vi "Main.vi"(11 "Module Admin":refnum<class "Delacor_lib_QMH_Module Admin.lvclass">) -> ()   [LabVIEW 2024, in "IOLink.lvlib"]
doc: "This template is based off of the Queued Message Handler design pattern and the Queued Message Handler project template that ships with LabVIEW.\n\nThe main difference is that the queue is private to this module and communication between modules is performed via Broadcast and Request events.\n\nRequest events are wrapped in public API methods and are handled in the Event Handling Loop (EHL) of this VI. Any module can register for Broadcast events sent by this module. The EHL generates messages based on user interface actions.\n\nThe Message Handling Loop (MHL) processes messages generated by the EHL, or by other messages. The messages are string values, so new messages can be added easily to the Message Cases case structure in the MHL. Each message cluster can also provide an optional value for Message Data, which is a variant that can be converted to whatever message-specific data is required.\n_____\nBased on DQMH Project Template 7.0.0.1280."
uses:
  IOLink.lvlib
  <vilib>/Delacor/Delacor QMH/Libraries/Module Admin_class/Delacor_lib_QMH_Module Admin.lvclass
  Module Data--cluster.ctl
  <vilib>/NI/Modbus Library/API/Master/Modbus Master.lvclass
  Start IOL Data Acquisition (Reply Payload)--cluster.ctl
  <vilib>/Delacor/Delacor QMH/Libraries/Message Queue_class/Delacor_lib_QMH_Message Queue.lvclass/Delacor_lib_QMH_Message Queue.ctl
  Stop Argument--cluster.ctl
  <vilib>/Delacor/Delacor QMH/Libraries/Module Admin_class/Delacor_lib_QMH_Module Admin.lvclass/Delacor_lib_QMH_Module Admin.ctl
  <vilib>/Utility/miscctls.llb/LVPointTypeDef.ctl
  <vilib>/Delacor/Delacor QMH/Libraries/Message Queue_class/Delacor_lib_QMH_Enqueue Message (Single).vi
  <vilib>/Delacor/Delacor QMH/Libraries/Module Admin_class/Delacor_lib_QMH_Get External Launch.vi
  <vilib>/NI/Modbus Library/API/Wrapper/Create TCP Master.vi
  <vilib>/Delacor/Delacor QMH/Libraries/Message Queue_class/Delacor_lib_QMH_Message Queue.lvclass
  <vilib>/NI/Modbus Library/API/Wrapper/API Main.lvlib
panel:
  out "map out":map{string, dbl}(c390)
  out "X5-8 Invalid Data":bool[](array[boolean])
  out "X5-8 Not Connected":bool[](array[boolean])
  out "X1-4 Invalid Data":bool[](array[boolean])
  out "X1-4 Not Connected":bool[](array[boolean])
  out "error out":errorcluster
  out "Status":string
  in  "Simulate MHL Error":bool
  in  "Simulate EHL Error":bool
  # "This template is for the DQMH framework. See the block diagram for more information on how to use this template."
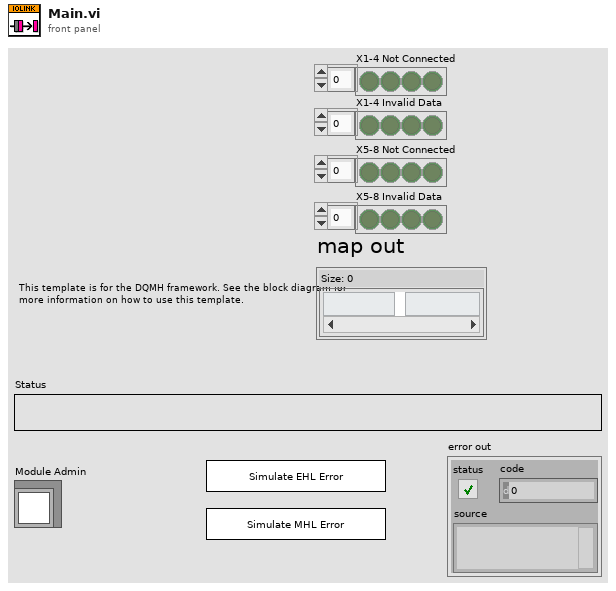
[diagram p1: front panel]
types:
  T1 = typedef "IOLink.lvlib/Request Events--cluster.ctl" = cluster{"Stop Module":refnum<user-event>, "Show Panel":refnum<user-event>, "Hide Panel":refnum<user-event>, "Get Module Execution Status":refnum<user-event>, "Show Diagram":refnum<user-event>, "Start IOL Data Acquisition":refnum<user-event>}
  T2 = typedef "IOLink.lvlib/Module Data--cluster.ctl" = cluster{"Status":string, "TCP master instance":refnum<class "Modbus Master.lvclass">}
  T3 = typedef "IOLink.lvlib/Start IOL Data Acquisition (Reply Payload)--cluster.ctl" = cluster{"error":errorcluster}
  T4 = enum32{"invalid lock state", "Not Locked", "Locked (No Password)", "Password-protected"}
  T5 = typedef "IOLink.lvlib/Stop Argument--cluster.ctl" = cluster{"Origin":string, "Exit via Stop Module Req?":bool, "Wait for Module to stop?":bool}
  T6 = typedef "LVPointTypeDef.ctl" = cluster{"Horizontal":i16, "Vertical":i16}
  T7 = enum32{"Invalid", "Standard", "Closed", "Hidden", "Minimized", "Maximized"}
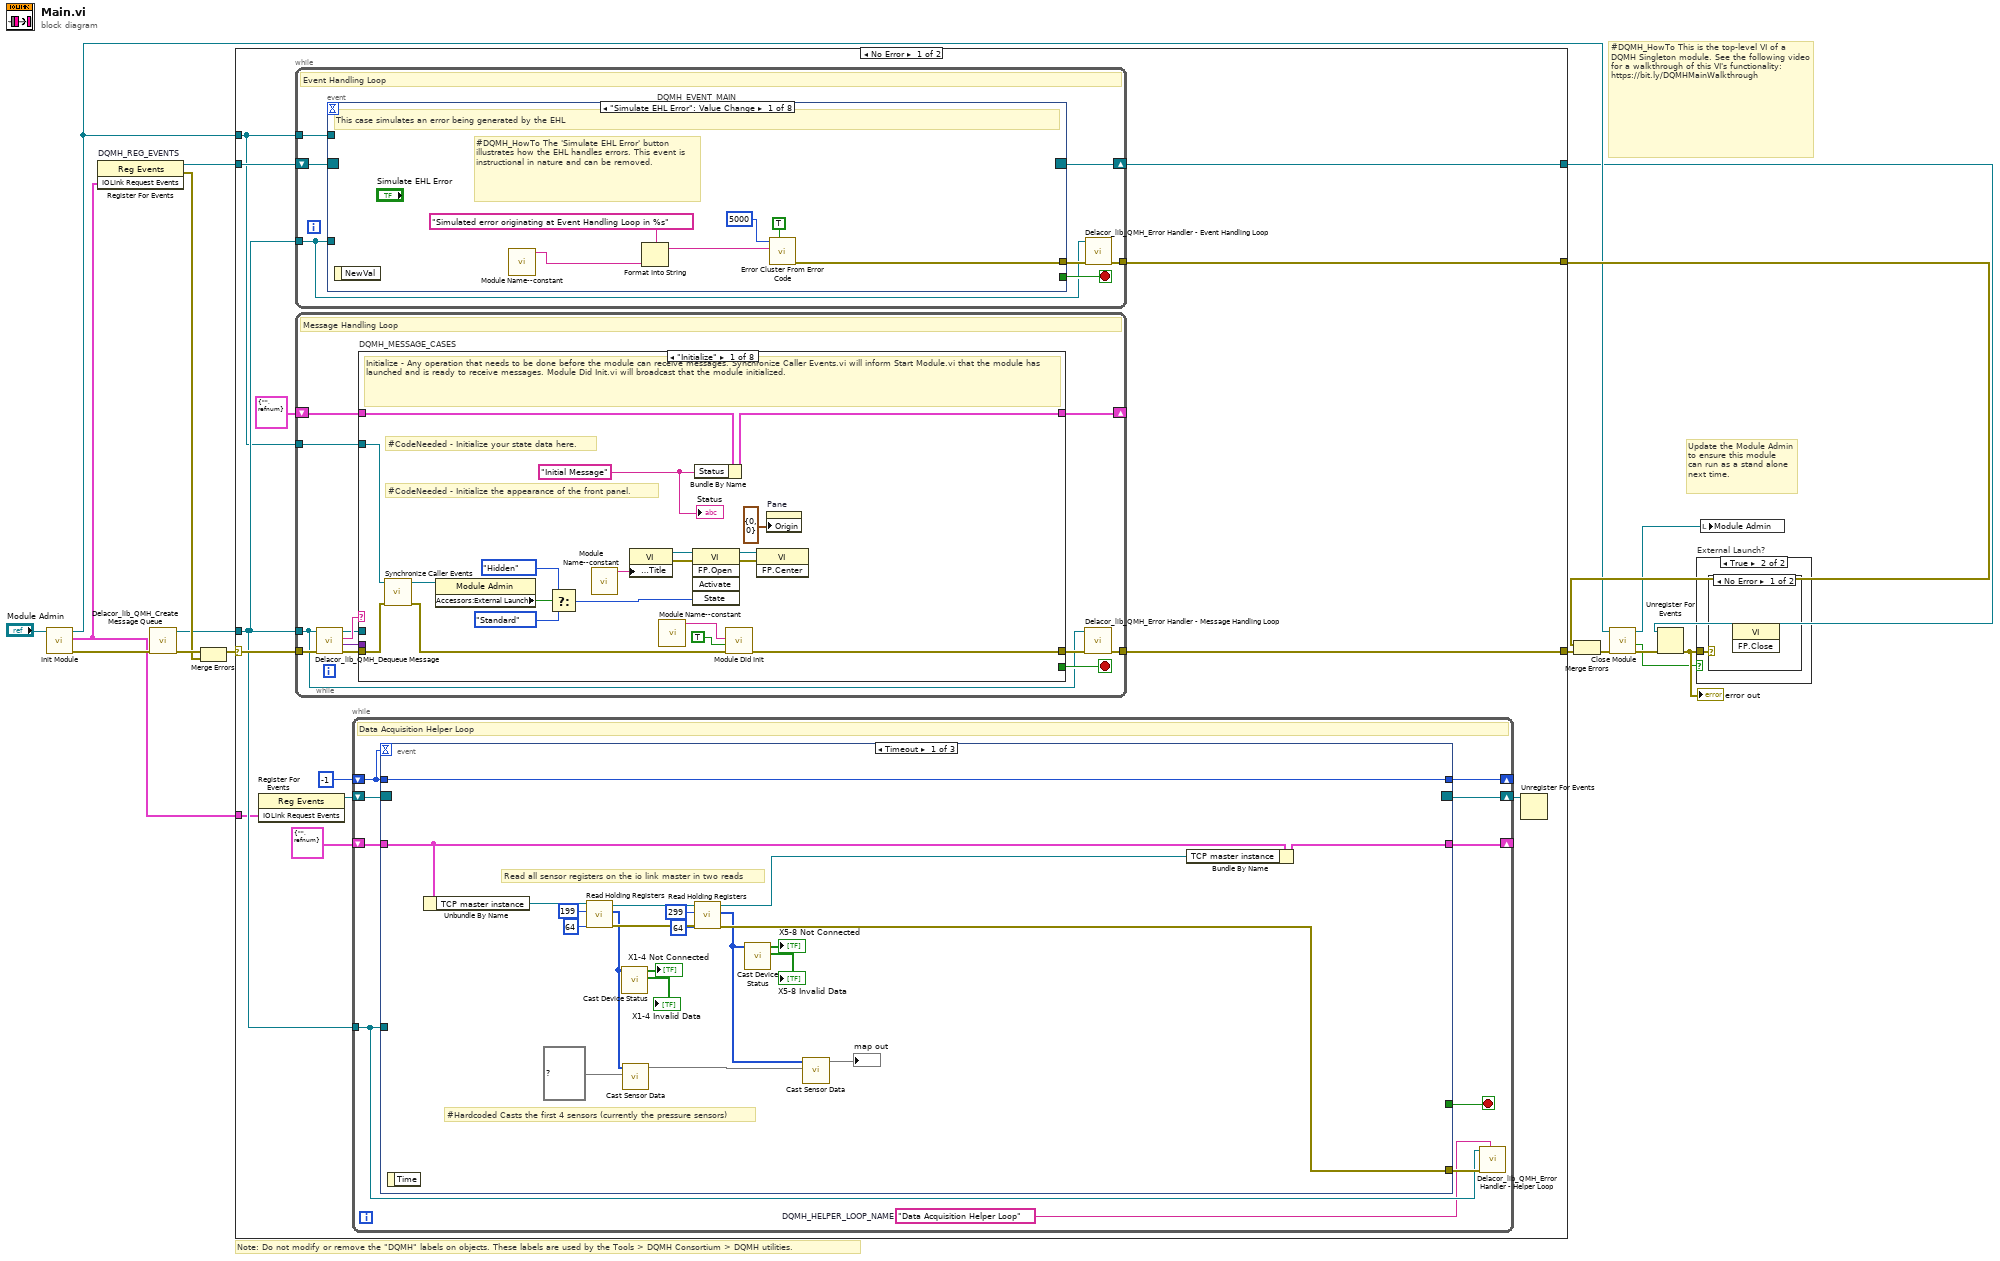
[diagram p0: block diagram]
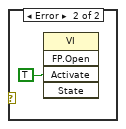
[diagram p3: hidden frame]
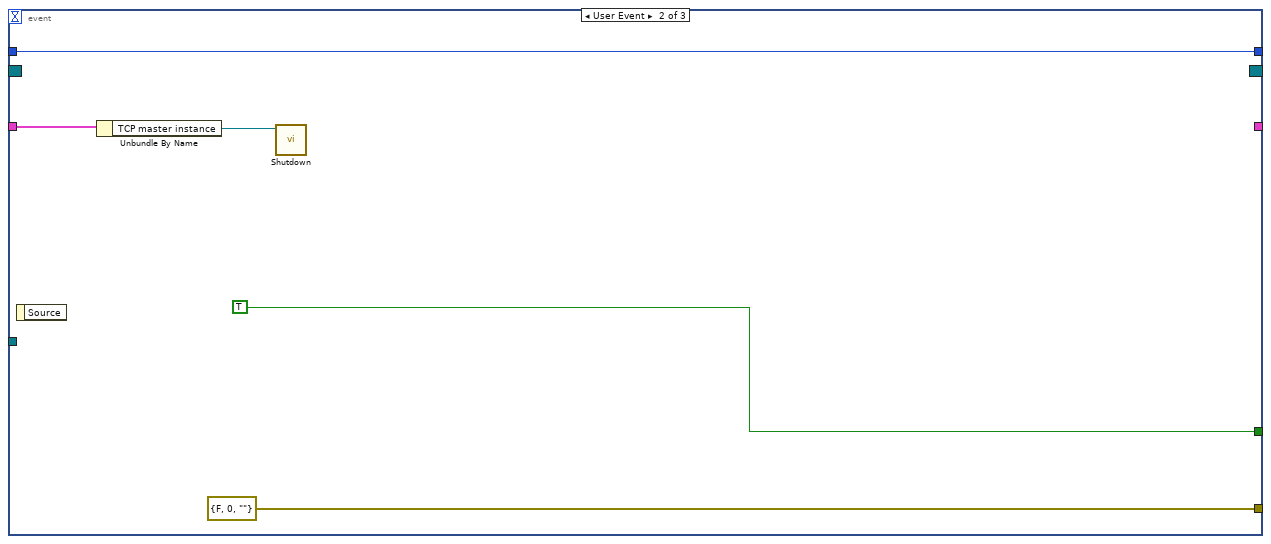
[diagram p4: hidden frame]
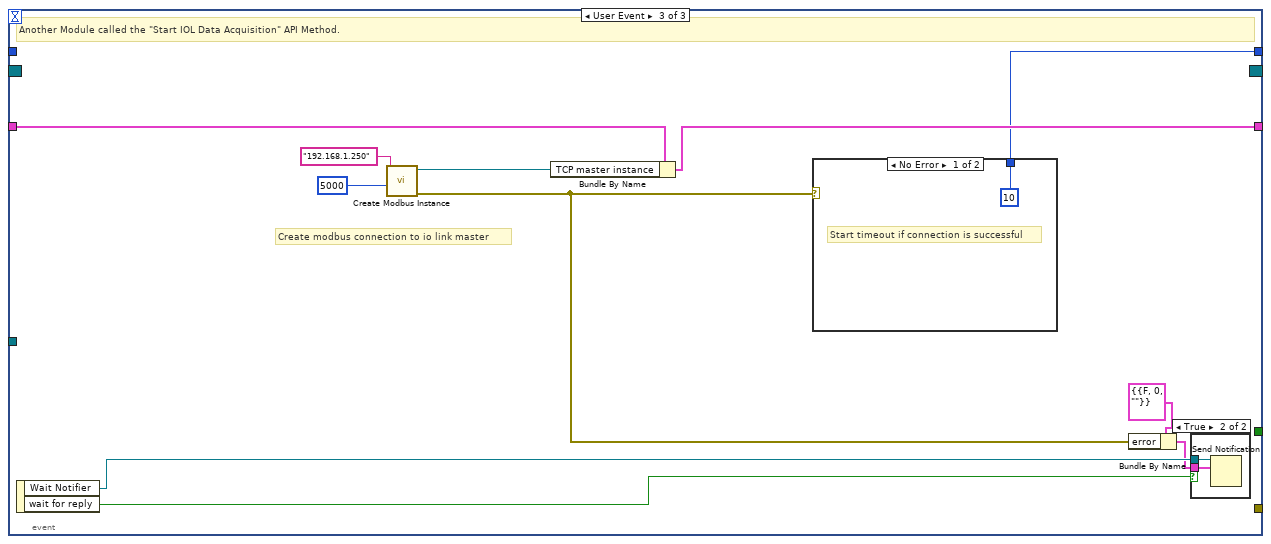
[diagram p5: hidden frame]
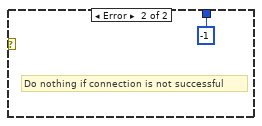
[diagram p6: hidden frame]
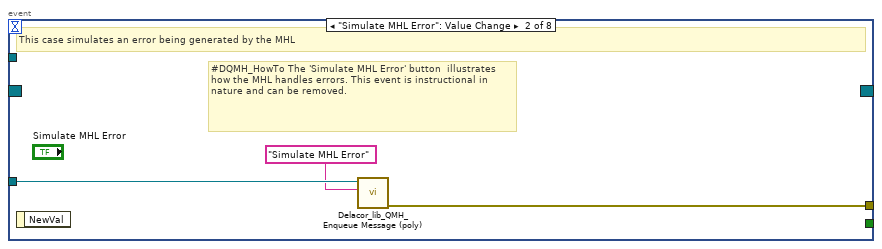
[diagram p8: hidden frame]
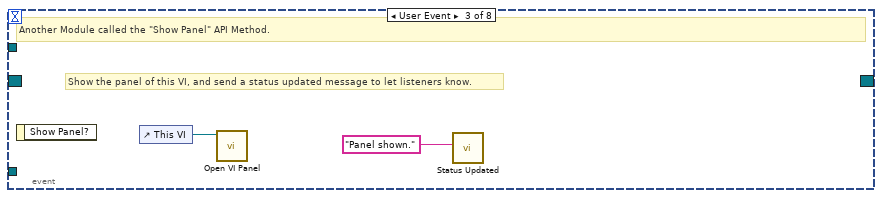
[diagram p9: hidden frame]
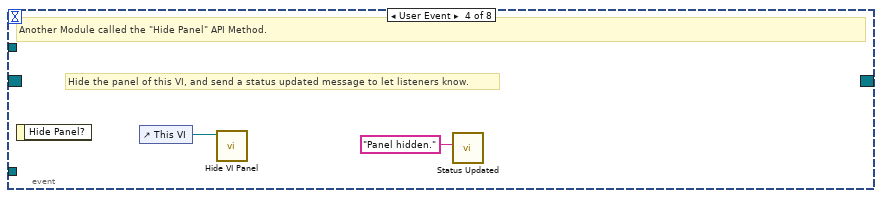
[diagram p10: hidden frame]
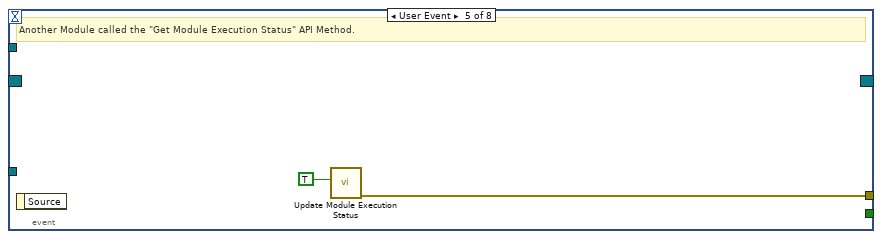
[diagram p11: hidden frame]
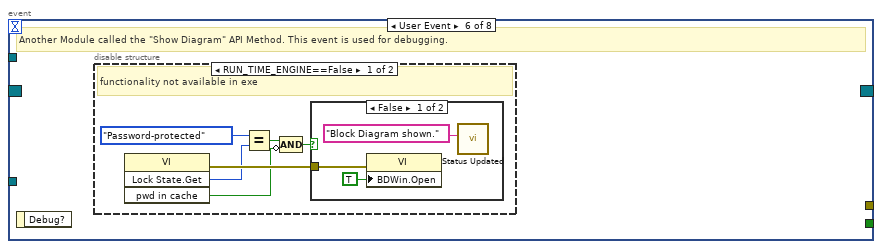
[diagram p12: hidden frame]
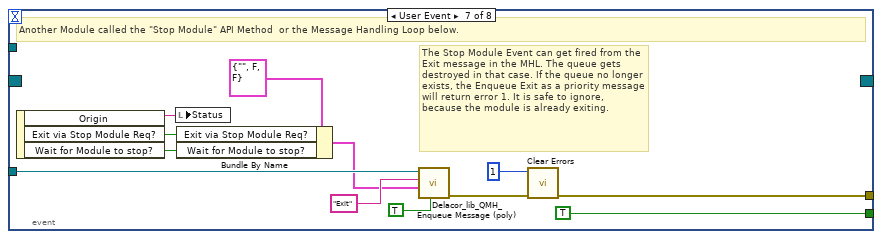
[diagram p15: hidden frame]
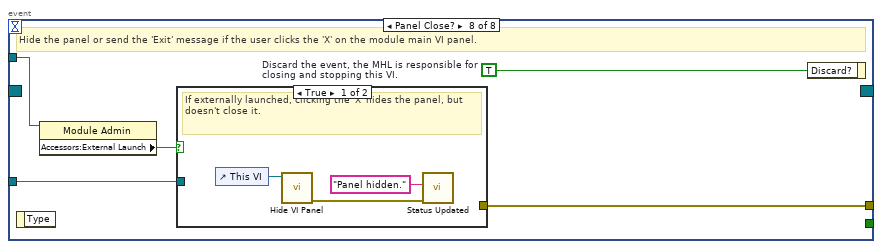
[diagram p16: hidden frame]
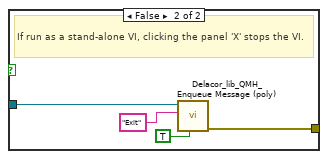
[diagram p17: hidden frame]
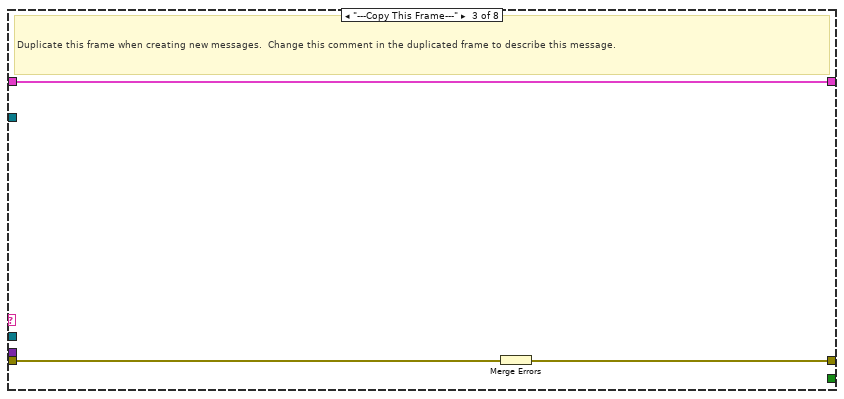
[diagram p19: hidden frame]
diagram:
  # "#DQMH_HowTo This is the top-level VI of a DQMH Singleton module. See the following video for a walkthrough of this VI's functionality: https://bit.ly/DQMHMainWalkthrough"
  # "Note: Do not modify or remove the \"DQMH\" labels on objects. These labels are used by the Tools > DQMH Consortium > DQMH utilities."
  # "Update the Module Admin to ensure this module can run as a stand alone next time."
  n1 = call "Init Module.vi"("Singleton Module Admin in"="Module Admin") -> ("error out"=w16:errorcluster, "IOLink Request Events"=w1:T1, "Singleton Module Admin out"=w8:refnum<class "Delacor_lib_QMH_Module Admin.lvclass">)  [unwired: 8 in]
  n2 = register-events "DQMH_REG_EVENTS"(w1) -> (reference out=w6:refnum<event-registration>, error out=w9:errorcluster)  [unwired: 2 in]
  n3 = call <vilib>:"Delacor_lib_QMH_Create Message Queue.vi"("error in"=w16) -> ("error out"=w11:errorcluster, "Message Queue"=w5:refnum<class "Delacor_lib_QMH_Message Queue.lvclass">)  [unwired: 9 in]
  n4 = Merge Errors(w11, w9) -> (w10:errorcluster)
  n5 = case shown="No Error" w10 {
    selector: w10 -> [w28 w234]
    tunnel: [w30 w233] -> w17
    tunnel: [w27 w232] -> w7
    tunnel: w6 -> [w25 w232]
    tunnel: w5 -> [w24 w227]
    tunnel: [w29 _] -> w14
    tunnel: w8 -> [w23 w228]
    tunnel: w1 -> [w22 _]
    frame No Error {
      n6 = register-events ("DQMH_HELPER_REGFOREVENTS")(w22) -> (reference out=w20:refnum<event-registration>)  [unwired: 2 in, 1 out]
      n7 = while {
        tunnel: w24 -> [w82]
        shift-right: [w85] -> w27
        shift-left: w25 -> [w86]
        tunnel: [w87] -> w29
        tunnel: w23 -> [w83]
        stop <- w84 stop-if-true
        # "Event Handling Loop"
        n8 = event "DQMH_EVENT_MAIN" shown="[0] \"Simulate EHL Error\": Value Change" {
          selector: w86 -> [_ _ _ _ _ _ _ _]
          dyn-events: [_ _ _ _ _ _ _ _] -> w85
          timeout: _ -> [_ _ _ _ _ _ _ _]
          tunnel: [_ _ _ _ _ _ TRUE ("Discard?") _] -> w84
          tunnel: w82 -> [_ w96 _ _ _ _ w120 w127]
          tunnel: [w94 w97 _ _ w103 _ w123 w129] -> w88
          tunnel: w83 -> [_ _ _ _ _ _ _ w126]
          event "Simulate EHL Error": Value Change {
            # "#DQMH_HowTo The 'Simulate EHL Error' button  illustrates how the EHL handles errors. This event is instructional in nature and can be removed."
            # "This case simulates an error being generated by the EHL"
            n9 = event-data() -> ()  [unwired: 1 in, 1 out]
            n10 = call "Module Name--constant.vi"() -> ("Module Name"=w91:string)  [unwired: 11 in]
            n11 = Format Into String(format string="Simulated error originating at Event Handling Loop in %s", w91) -> (resulting string=w92:string)  [unwired: 2 in, 1 out]
            n12 = call <vilib>:"Error Cluster From Error Code.vi"("show call chain? (False)"=TRUE, "error message (\"\")"=w92, "error code (0)"=5000) -> ("error out"=w94:errorcluster)  [unwired: 6 in]
          }
          event "Simulate MHL Error": Value Change {
            # "#DQMH_HowTo The 'Simulate MHL Error' button  illustrates how the MHL handles errors. This event is instructional in nature and can be removed."
            # "This case simulates an error being generated by the MHL"
            n13 = event-data() -> ()  [unwired: 1 in, 1 out]
            n14 = call-poly <vilib>:"Delacor_lib_QMH_Enqueue Message (poly).vi"("Message"="Simulate MHL Error", "Message Queue in"=w96) -> ("error out"=w97:errorcluster)  [unwired: 8 in, 1 out]
          }
          event User Event {
            # "Show the panel of this VI, and send a status updated message to let listeners know."
            # "Another Module called the \"Show Panel\" API Method."
            n15 = event-data() -> ()  [unwired: 1 in, 1 out]
            n16 = control-ref of="This VI"() -> (w99:refnum<vi>)
            n17 = call "Open VI Panel.vi"("VI"=w99) -> ()  [unwired: 10 in, 1 out]
            n18 = call "Status Updated.vi"("Status"="Panel shown." ("format string")) -> ()  [unwired: 10 in, 1 out]
          }
          event User Event {
            # "Hide the panel of this VI, and send a status updated message to let listeners know."
            # "Another Module called the \"Hide Panel\" API Method."
            n19 = event-data() -> ()  [unwired: 1 in, 1 out]
            n20 = control-ref of="This VI"() -> (w101:refnum<vi>)
            n21 = call "Hide VI Panel.vi"("VI"=w101) -> ()  [unwired: 10 in, 1 out]
            n22 = call "Status Updated.vi"("Status"="Panel hidden." ("format string")) -> ()  [unwired: 10 in, 1 out]
          }
          event User Event {
            # "Another Module called the \"Get Module Execution Status\" API Method."
            n23 = event-data() -> ()  [unwired: 1 in, 1 out]
            n24 = call "Update Module Execution Status.vi"("Running?"=TRUE) -> ("error out"=w103:errorcluster)  [unwired: 10 in]
          }
          event User Event {
            # "Another Module called the \"Show Diagram\" API Method. This event is used for debugging."
            n25 = event-data() -> ()  [unwired: 1 in, 1 out]
            n26 = disable-structure shown="RUN_TIME_ENGINE==False" {
              frame condition #0 (active) {
                # "functionality not available in exe"
                n27 = invoke class="VI" method="Lock State.Get"() -> (error out=w109:errorcluster, "Get Lock State"=w108:T4, "pwd in cache"=w105:bool)  [unwired: 4 in, 1 out]
                n28 = Equal?(x=T4."Password-protected", y=w108) -> (x = y?=w106:bool)
                n29 = Compound Arithmetic op=AND(w106, invert w105) -> (w104:bool)
                n30 = case shown="False" w104 {
                  tunnel: w109 -> [w112 _]
                  frame False {
                    n31 = property class="VI"(error in=w112, "BDWin.Open"=TRUE ("Block Diagram Window:Open")) -> ()  [unwired: 1 in, 2 out]
                    n32 = call "Status Updated.vi"("Status"="Block Diagram shown." ("format string")) -> ()  [unwired: 10 in, 1 out]
                  }
                  frame True {
                    # "Password-protected VI, and the password is not in the cache. Do not show the diagram."
                  }
                }
              }
              frame condition #1 {
              }
            }
          }
          event User Event {
            # "The Stop Module Event can get fired from the Exit message in the MHL. The queue gets destroyed in that case. If the queue no longer exists, the Enqueue Exit as a priority message will return error 1. It is safe to ignore, because the module is already exiting."
            # "Another Module called the \"Stop Module\" API Method  or the Message Handling Loop below."
            n33 = event-data() -> ("Origin"=w119:string, "Exit via Stop Module Req?"=w115:bool, "Wait for Module to stop?"=w114:bool)  [unwired: 1 in]
            n34 = local write "Status"(w119) -> ()
            n35 = Bundle By Name(cluster=T5 {"Origin"="", "Exit via Stop Module Req?"=FALSE, "Wait for Module to stop?"=FALSE} ("Stop Argument"), "Exit via Stop Module Req?"=w115, "Wait for Module to stop?"=w114) -> (w113:T5)
            n36 = call-poly <vilib>:"Delacor_lib_QMH_Enqueue Message (poly).vi"("Priority Message? (F)"=TRUE, "Message Data"=w113, "Message"="Exit", "Message Queue in"=w120) -> ("error out"=w124:errorcluster)  [unwired: 6 in, 1 out]
            n37 = call <vilib>:"Clear Errors.vi"("error in (no error)"=w124, "specific error code to clear (0: all)"=1) -> ("error out"=w123:errorcluster)  [unwired: 4 in, 1 out]
          }
          event Panel Close? {
            w128 = TRUE  # Discard the event, the MHL is responsible for closing and stopping this VI.
            # "Hide the panel or send the 'Exit' message if the user clicks the 'X' on the module main VI panel."
            n38 = event-data() -> ()  [unwired: 1 in, 1 out]
            n39 = property class="Module Admin"(reference=w126) -> ("Accessors:External Launch"=w125:bool)  [unwired: 1 in, 2 out]
            n40 = case shown="True" w125 {
              tunnel: w127 -> [_ w135]
              tunnel: [_ w136] -> w129
              frame True {
                # "If externally launched, clicking the 'X' hides the panel, but doesn't close it."
                n41 = control-ref of="This VI"() -> (w132:refnum<vi>)
                n42 = call "Hide VI Panel.vi"("VI"=w132) -> ("error out"=w130:errorcluster)  [unwired: 10 in]
                n43 = call "Status Updated.vi"("error in"=w130, "Status"="Panel hidden." ("format string")) -> ()  [unwired: 9 in, 1 out]
              }
              frame False {
                # "If run as a stand-alone VI, clicking the panel 'X' stops the VI."
                n44 = call-poly <vilib>:"Delacor_lib_QMH_Enqueue Message (poly).vi"("Priority Message? (F)"=TRUE, "Message"="Exit", "Message Queue in"=w135) -> ("error out"=w136:errorcluster)  [unwired: 7 in, 1 out]
              }
            }
            n45 = event-data("Discard?"=w128) -> ()  [unwired: 1 in, 1 out]
          }
        }
        n46 = call-dynamic "Delacor_lib_QMH_Error Handler - Event Handling Loop.vi"("error in"=w88, "Message Queue in"=w82) -> ("dup error in"=w87:errorcluster)  [unwired: 8 in, 1 out]
      }
      n47 = while {
        tunnel: w24 -> [w137]
        shift-right: [w143] -> _
        shift-left: T2 {"Status"="", "TCP master instance"=refnum} ("Data Cluster") -> [w144]
        tunnel: w28 -> [w147]
        tunnel: [w145] -> w30
        tunnel: w23 -> [w138]
        stop <- w142 stop-if-true
        # "Message Handling Loop"
        n48 = call-dynamic "Delacor_lib_QMH_Dequeue Message.vi"("error in"=w147, "Message Queue in"=w137) -> ("error out"=w146:errorcluster, "Message Data"=w140:variant, "Message"=w141:string, "Message Queue out"=w139:refnum<class "Delacor_lib_QMH_Message Queue.lvclass">)  [unwired: 6 in]
        n49 = case "DQMH_MESSAGE_CASES" shown="\"Initialize\"" w141 {
          selector: w141 -> [_ _ _ _ _ _ _ w222]
          tunnel: w139 -> [_ _ _ _ _ w188 w210 _]
          tunnel: w146 -> [w166 w170 w173 w175 w184 w195 w216 w225]
          tunnel: [w164 w170 w172 w175 w183 w191 w211 w226] -> w148
          tunnel: w144 -> [w155 w169 w171 w174 w181 w190 w209 w223]
          tunnel: [w154 w169 w171 w174 w181 w190 w209 w223] -> w143
          tunnel: [_ _ _ _ _ _ w208 _] -> w142
          tunnel: w140 -> [_ _ _ _ _ w189 w207 _]
          tunnel: w138 -> [w156 _ _ _ _ w187 w202 _]
          frame "Initialize" {
            w150 = "Initial Message" ("Initial Message")
            # "#CodeNeeded - Initialize the appearance of the front panel."
            # "#CodeNeeded - Initialize your state data here."
            # "Initialize - Any operation that needs to be done before the module can receive messages. Synchronize Caller Events.vi will inform Start Module.vi that the module has launched and is ready to receive messages. Module Did Init.vi will broadcast that the module initialized."
            n50 = call "Synchronize Caller Events.vi"("error in"=w166, "Singleton Module Admin in"=w156) -> ("error out"=w165:errorcluster, "Singleton Module Admin out"=w151:refnum<class "Delacor_lib_QMH_Module Admin.lvclass">)  [unwired: 8 in]
            n51 = property class="Module Admin"(reference=w151) -> ("Accessors:External Launch"=w160:bool)  [unwired: 1 in, 2 out]
            n52 = Select(t=T7."Hidden" ("State"), s=w160, f=T7."Standard" ("State")) -> (s? t:f=w157:T7)
            n53 = call "Module Name--constant.vi"() -> ("Module Name"=w163:string)  [unwired: 11 in]
            n54 = property class="VI"("Front Panel.Title"=w163) -> (reference out=w162:refnum<vi>, error out=w168:errorcluster)  [unwired: 2 in]
            n55 = call "Module Name--constant.vi"() -> ("Module Name"=w152:string)  [unwired: 11 in]
            n56 = invoke class="VI" method="FP.Open"(reference=w162, error in=w168, "State"=w157) -> (reference out=w161:refnum<vi>, error out=w167:errorcluster)  [unwired: 2 in, 3 out]
            n57 = Bundle By Name(cluster=w155, "Status"=w150) -> (w154:T2)
            n58 = call "Module Did Init.vi"("error in"=w165, "Initialized?"=TRUE, "Origin"=w152) -> ("error out"=w164:errorcluster)  [unwired: 8 in]
            n59 = invoke class="VI" method="FP.Center"(reference=w161, error in=w167) -> ()  [unwired: 1 in, 3 out]
            n60 = property on="Pane" class="Pane"("Origin"=T6 {"Horizontal"=0, "Vertical"=0}) -> ()  [unwired: 2 in, 2 out]
            "Status" <- w150
          }
          frame "---Module Specific---" {
            # "Separator -- The following cases handle messages specific to this Module."
          }
          frame "---Copy This Frame---" {
            # "Duplicate this frame when creating new messages.  Change this comment in the duplicated frame to describe this message."
            n61 = Merge Errors(w173) -> (w172:errorcluster)
          }
          frame "---Exit and Error Handling---" {
            # "Separator - The following cases handle errors and exit messages."
          }
          frame "Simulate MHL Error" {
            # "#DQMH_HowTo The 'Simulate MHL Error' button  illustrates how the MHL handles errors. This event is instructional in nature and can be removed."
            # "Simulate an error occurring at the MHL"
            n62 = call "Module Name--constant.vi"() -> ("Module Name"=w177:string)  [unwired: 11 in]
            n63 = Format Into String(format string="Simulated error originating at Message Handling Loop in %s", w177) -> (resulting string=w178:string)  [unwired: 2 in, 1 out]
            n64 = call <vilib>:"Error Cluster From Error Code.vi"("show call chain? (False)"=TRUE, "error message (\"\")"=w178, "error code (0)"=5001) -> ("error out"=w182:errorcluster)  [unwired: 6 in]
            n65 = Merge Errors(w184, w182) -> (w183:errorcluster)
          }
          frame "Error" {
            # "#CodeRecommended - If the module is running in standalone mode (External Launch = FALSE), this code will pop up an error dialog and call the 'Exit' message if an error occurs. Add more fine-grained error management here."
            # "Error - Check the error message data and respond accordingly. This message is sent by the \"Error Handler\" VIs at the end of each loop in this application."
            n66 = property class="Module Admin"(reference=w187) -> ("Accessors:External Launch"=w186:bool)  [unwired: 1 in, 2 out]
            n67 = Variant To Data(error in=w195, type=errorcluster {"status"=FALSE, "code"=0, "source"=""} ("error constant"), Variant=w189) -> (data=w185:errorcluster, error out=w193:errorcluster)
            n68 = local write "error out"(w185) -> ()
            n69 = call "Error Reported.vi"("Error"=w185) -> ()  [unwired: 10 in, 1 out]
            n70 = case shown="False" w186 {
              tunnel: [w200 _] -> w192
              tunnel: w188 -> [w198 _]
              tunnel: w185 -> [w199 _]
              frame False {
                n71 = disable-structure shown="Default" {
                  disable-tunnel: w199 -> [w201 _]
                  frame condition #0 (active) {
                    # "If the module is running standalone, then pop up an error dialog and call the \"Exit\" message."
                    n72 = call <vilib>:"Simple Error Handler.vi"("error in (no error)"=w201) -> ()  [unwired: 4 in, 5 out]
                  }
                  frame condition #1 {
                    # "To prevent the Simple Error Handler VI from being loaded (e.g. when deploying to a Real-Time target), add the Conditional Disable Symbol \"DQMH_Disable_SEH\" to your project and set it to TRUE."
                  }
                }
                n73 = call-poly <vilib>:"Delacor_lib_QMH_Enqueue Message (poly).vi"("Priority Message? (F)"=TRUE, "Message"="Exit", "Message Queue in"=w198) -> ("error out"=w200:errorcluster)  [unwired: 7 in, 1 out]
              }
              frame True {
                # "If the module was launched externally, calling the Error Reported broadcast VI is the only action performed by the \"Error\" message. The module's caller can then process the error appropriately."
              }
            }
            n74 = Merge Errors(w193, w192) -> (w191:errorcluster)
          }
          frame "Exit" {
            w206 = 91  # 91: not all Exit messages will have an argument
            w208 = TRUE  # Stop the VI
            # "Release the message queue reference"
            # "#CodeNeeded - Add any required cleanup code here."
            # "Exit - Exit the application."
            n75 = Variant To Data(error in=w216, type=T5 {"Origin"="", "Exit via Stop Module Req?"=FALSE, "Wait for Module to stop?"=FALSE} ("Stop Argument"), Variant=w207) -> (data=w204:T5, error out=w213:errorcluster)
            n76 = call <vilib>:"Clear Errors.vi"("error in (no error)"=w213, "specific error code to clear (0: all)"=w206) -> ("error out"=w215:errorcluster)  [unwired: 4 in, 1 out]
            n77 = control-ref of="This VI"() -> (w203:refnum<vi>)
            n78 = call-dynamic "Delacor_lib_QMH_Release Message Queue.vi"("error in"=w215, "Message Queue"=w210) -> ("error out"=w214:errorcluster)  [unwired: 9 in]
            n79 = call "Handle Exit.vi"("Stop Argument"=w204, "Admin in"=w202, "VI reference"=w203) -> ("error out"=w212:errorcluster)  [unwired: 7 in, 1 out]
            n80 = Merge Errors(w214, w212) -> (w211:errorcluster)
            n81 = call "Error Reported.vi"("Error"=w211) -> ()  [unwired: 10 in, 1 out]
          }
          frame Default {
            # "'Default' case only runs if there is a message that isn't defined in any of the other cases.  Output a programming error."
            n82 = call "Module Name--constant.vi"() -> ("Module Name"=w221:string)  [unwired: 11 in]
            n83 = Format Into String(format string="The invalid message string \"%s\" was received in the Message Handling Loop for module \"%s\".", w222, w221) -> (resulting string=w217:string)  [unwired: 2 in, 1 out]
            n84 = call <vilib>:"Error Cluster From Error Code.vi"("show call chain? (False)"=TRUE, "error message (\"\")"=w217, "error code (0)"=1) -> ("error out"=w224:errorcluster)  [unwired: 6 in]
            n85 = Merge Errors(w225, w224) -> (w226:errorcluster)
          }
        }
        n86 = call-dynamic "Delacor_lib_QMH_Error Handler - Message Handling Loop.vi"("error in"=w148, "Message Queue in"=w137) -> ("dup error in"=w145:errorcluster)  [unwired: 8 in, 1 out]
      }
      n87 = while "DQMH_HELPER_LOOP" {
        shift-right: [w40] -> _
        shift-left: -1 -> [w39]
        shift-right: [w37] -> w21
        shift-left: w20 -> [w38]
        tunnel: w24 -> [w34]
        shift-right: [w31] -> _
        shift-left: T2 {"Status"="", "TCP master instance"=refnum} ("Data Cluster") -> [w32]
        stop <- w36 stop-if-true
        w33 = "Data Acquisition Helper Loop"  # DQMH_HELPER_LOOP_NAME
        # "Data Acquisition Helper Loop"
        n88 = event "DQMH_HELPER_EVENT_STRUCTURE" shown="[0] Timeout" {
          selector: w38 -> [_ _ _]
          dyn-events: [_ _ _] -> w37
          timeout: w39 -> [_ _ _]
          tunnel: w39 -> [w61 w66 _]
          tunnel: [w61 w66 w67] -> w40
          tunnel: [_ TRUE _] -> w36
          tunnel: [w50 errorcluster {"status"=FALSE, "code"=0, "source"=""} ("error constant") _] -> w35
          tunnel: w34 -> [_ _ _]
          tunnel: w32 -> [w60 w63 w69]
          tunnel: [w52 _ w70] -> w31
          event Timeout {
            # "#Hardcoded Casts the first 4 sensors (currently the pressure sensors)"
            # "Read all sensor registers on the io link master in two reads"
            n89 = event-data() -> ()  [unwired: 1 in, 1 out]
            n90 = Unbundle By Name(w60) -> ("TCP master instance"=w59:refnum<class "Modbus Master.lvclass">)
            n91 = call-dynamic "Read Holding Registers.vi"("number of inputs"=u16 64, "starting address"=u16 199, "Modbus master in"=w59) -> ("error out"=w55:errorcluster, "register values"=w45:u16[], "Modbus master out"=w56:refnum<class "Modbus Master.lvclass">)  [unwired: 6 in]
            n92 = call "Cast Device Status.vi"("register values"=w45) -> ("Invalid Data"=→"X1-4 Invalid Data":bool[], "Connected"=→"X1-4 Not Connected":bool[])  [unwired: 9 in]
            n93 = call "Cast Sensor Data.vi"("Map"=map{string, dbl} {}, "register values"=w45) -> ("map out"=w42:map{string, dbl})  [unwired: 9 in]
            n94 = call-dynamic "Read Holding Registers.vi"("error in"=w55, "number of inputs"=u16 64, "starting address"=u16 299, "Modbus master in"=w56) -> ("error out"=w50:errorcluster, "register values"=w44:u16[], "Modbus master out"=w51:refnum<class "Modbus Master.lvclass">)  [unwired: 5 in]
            n95 = call "Cast Device Status.vi"("register values"=w44) -> ("Invalid Data"=→"X5-8 Invalid Data":bool[], "Connected"=→"X5-8 Not Connected":bool[])  [unwired: 9 in]
            n96 = call "Cast Sensor Data.vi"("Map"=w42, "register values"=w44) -> ("map out"=→"map out":map{string, dbl})  [unwired: 9 in]
            n97 = Bundle By Name(cluster=w60, "TCP master instance"=w51) -> (w52:T2)
          }
          event User Event {
            n98 = event-data() -> ()  [unwired: 1 in, 1 out]
            n99 = Unbundle By Name(w63) -> ("TCP master instance"=w62:refnum<class "Modbus Master.lvclass">)
            n100 = call-dynamic "Shutdown.vi"("Modbus master in"=w62) -> ()  [unwired: 10 in, 1 out]
          }
          event User Event {
            # "Create modbus connection to io link master"
            # "Another Module called the \"Start IOL Data Acquisition\" API Method."
            n101 = event-data() -> ("Wait Notifier"=w77:refnum<notifier>, "wait for reply"=w76:bool)  [unwired: 1 in]
            n102 = call-poly <vilib>:"Create Modbus Instance.vi"("connect timeout ms"=5000, "address"="192.168.1.250") -> ("error out"=w68:errorcluster, "TCP master instance"=w71:refnum<class "Modbus Master.lvclass">)  [unwired: 8 in]
            n103 = Bundle By Name(cluster=w69, "TCP master instance"=w71) -> (w70:T2)
            n104 = case shown="No Error" w68 {
              tunnel: [10 -1] -> w67
              frame No Error {
                # "Start timeout if connection is successful"
              }
              frame Error {
                # "Do nothing if connection is not successful"
              }
            }
            n105 = Bundle By Name(cluster=T3 {"error"={"status"=FALSE, "code"=0, "source"=""}} ("Start IOL Data Acquisition (Reply Payload)"), "error"=w68) -> (w75:T3)
            n106 = case "DQMH_FIRE_NOTIFIER" shown="True" w76 {
              tunnel: w77 -> [_ w81]
              tunnel: w75 -> [_ w80]
              frame False {
              }
              frame True {
                n107 = Send Notification(notification=w80, notifier=w81) -> ()  [unwired: 1 in, 2 out]
              }
            }
          }
        }
        n108 = call-dynamic "Delacor_lib_QMH_Error Handler - Helper Loop.vi"("Error Debug"=w33, "error in"=w35, "Message Queue in"=w34) -> ()  [unwired: 7 in, 2 out]
      }
      n109 = Unregister For Events(event registration refnum=w21) -> ()  [unwired: 1 in, 1 out]
    }
    frame Error {
      # "Synchronize Caller Events.vi will inform Start Module.vi that the module has launched and will let the code calling Start Module.vi register for broadcasts and would permit the caller receive the broadcast that an error occurred at launch time."
      n110 = call-dynamic "Delacor_lib_QMH_Release Message Queue.vi"("error in"=w234, "Message Queue"=w227) -> ("error out"=w233:errorcluster)  [unwired: 9 in]
      n111 = call "Synchronize Caller Events.vi"("Singleton Module Admin in"=w228) -> ("error out"=w235:errorcluster)  [unwired: 9 in, 1 out]
      n112 = call "Module Name--constant.vi"() -> ("Module Name"=w231:string)  [unwired: 11 in]
      n113 = Format Into String(format string="An error occurred during initialization. %s is no longer running.", w231) -> (resulting string=w229:string)  [unwired: 2 in, 1 out]
      n114 = Merge Errors(w233, w235) -> (w236:errorcluster)
      n115 = call "Error Reported.vi"("Additional Information"=w229, "Error"=w236) -> ()  [unwired: 9 in, 1 out]
    }
  }
  n116 = Merge Errors(w14, w17) -> (w13:errorcluster)
  n117 = call "Close Module.vi"("error in"=w13, "Module Admin in"=w8) -> ("error out"=w15:errorcluster, "External Launch"=w2:bool, "Module Admin out"=w3:refnum<class "Delacor_lib_QMH_Module Admin.lvclass">)  [unwired: 7 in]
  n118 = Unregister For Events(event registration refnum=w7, error in=w15) -> (error out=w12:errorcluster)
  "error out" <- w12
  n119 = case "External Launch?" shown="True" w2 {
    tunnel: w12 -> [_ w237]
    frame False {
    }
    frame True {
      n120 = case shown="No Error" w237 {
        frame No Error {
          n121 = invoke class="VI" method="FP.Close"() -> ()  [unwired: 3 in, 3 out]
        }
        frame Error {
          n122 = invoke class="VI" method="FP.Open"("Activate"=TRUE ("Activate?")) -> ()  [unwired: 4 in, 5 out]
        }
      }
    }
  }
  n123 = local write "Module Admin"(w3) -> ()
